vi "testRawXmlMultiLine.vi"(8 "error in (no error)":errorcluster, 11 "TestCase in":refnum<class "EasyXMLTest.lvclass">) -> (0 "error out":errorcluster, 3 "TestCase out":refnum<class "EasyXMLTest.lvclass">)   [LabVIEW 2013, in "EasyXMLTest.lvclass"]
doc: "Verify that error in is not overwritten"
uses:
  EasyXMLTest.lvclass
  <userlib>/_OpenG.lib/string/string.llb/Convert EOLs (String)__ogtk.vi
panel:
  out "data":string
  out "Produced Data":variant
  out "Input Data":variant
  out "XML String":string
  out "Generated XML String":string
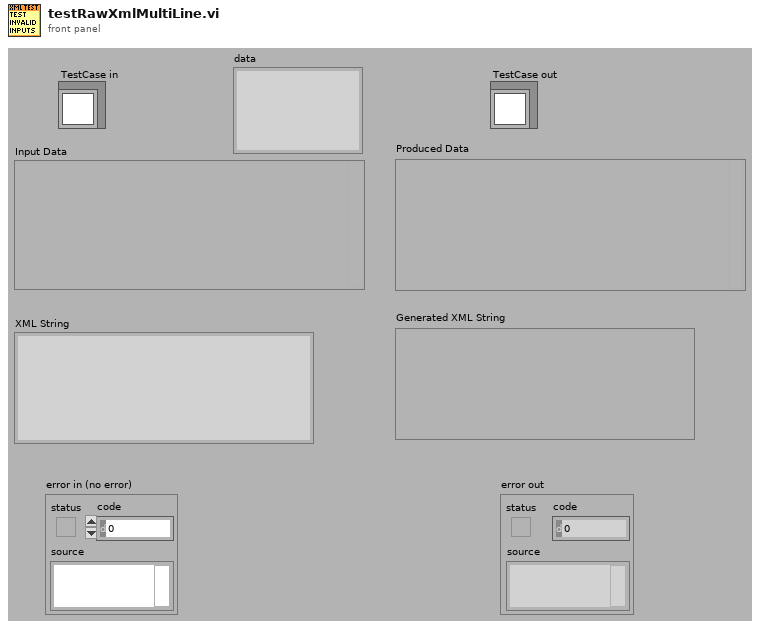
[diagram p1: front panel]
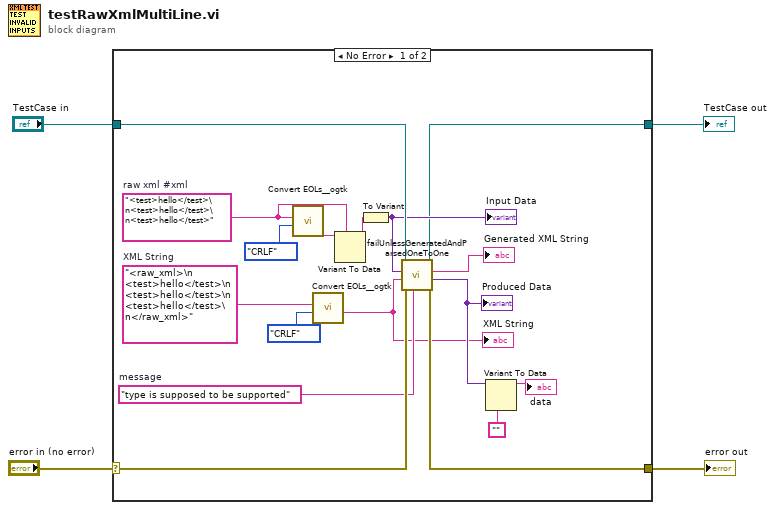
[diagram p0: block diagram]
diagram:
  n1 = case shown="No Error" "error in (no error)" {
    selector: "error in (no error)" -> [w20 w23]
    tunnel: [w16 w23] -> w2
    tunnel: [w15 w22] -> w1
    tunnel: "TestCase in" -> [w21 w22]
    frame No Error {
      w7 = "<test>hello</test>\n<test>hello</test>\n<test>hello</test>"  # raw xml #xml
      w14 = "<raw_xml>\n  <test>hello</test>\n  <test>hello</test>\n  <test>hello</test>\n</raw_xml>"  # XML String
      w19 = "type is supposed to be supported"  # message
      n2 = call-poly <userlib>:"Convert EOLs__ogtk.vi"("Convert to:"=enum16{"CR", "LF", "CRLF"}."CRLF", "String in"=w7) -> ("String out"=w6:string)  [unwired: 9 in]
      n3 = call-poly <userlib>:"Convert EOLs__ogtk.vi"("Convert to:"=enum16{"CR", "LF", "CRLF"}."CRLF", "String in"=w14) -> ("String out"=w10:string)  [unwired: 9 in]
      "XML String" <- w10
      n4 = Variant To Data(type=w7, Variant=w6) -> (data=w5:string)  [unwired: 1 in, 1 out]
      n5 = To Variant(anything=w5) -> (Variant=w18:variant)
      "Input Data" <- w18
      n6 = call "failUnlessGeneratedAndParsedOneToOne.vi"("message (\"\")"=w19, "error in"=w20, "XML String"=w10, "Data"=w18, "EasyXMLTest in"=w21) -> ("error out"=w16:errorcluster, "Produced Data"=w13:variant, "Generated XML String"=→"Generated XML String":string, "EasyXMLTest out"=w15:refnum<class "EasyXMLTest.lvclass">)  [unwired: 3 in]
      "Produced Data" <- w13
      n7 = Variant To Data(type="", Variant=w13) -> (data=→"data":string)  [unwired: 1 in, 1 out]
    }
    frame Error {
    }
  }
  "error out" <- w2
  "TestCase out" <- w1
